vi "Copy exp data.vi"(8 "error in (no error)":errorcluster, 9 "selected wavelengths":dbl[](array[numeric])=[550.0, 640.0, 680.0, 720.0, 780.0, 800.0], 10 "ItemTag":string, 11 "Control-Client in":refnum<class "Control-Client.lvclass">) -> (0 "error out":errorcluster, 3 "Control-Client out":refnum<class "Control-Client.lvclass">)   [LabVIEW 2018, in "Control-Client.lvclass"]
uses:
  Control-Client.lvclass
  C:/Users/Sergey Denisov/Documents/REPS/TRANCON/Classes/GeneralFunctionality/GeneralFunctionality.lvclass
  GeneralFunctionality/GeneralFunctionality.lvclass/GeneralFunctionality.ctl
  Config/Config.lvclass
  Experiments/Experiment.lvclass
  GeneralFunctionality/GeneralFunctionality.lvclass
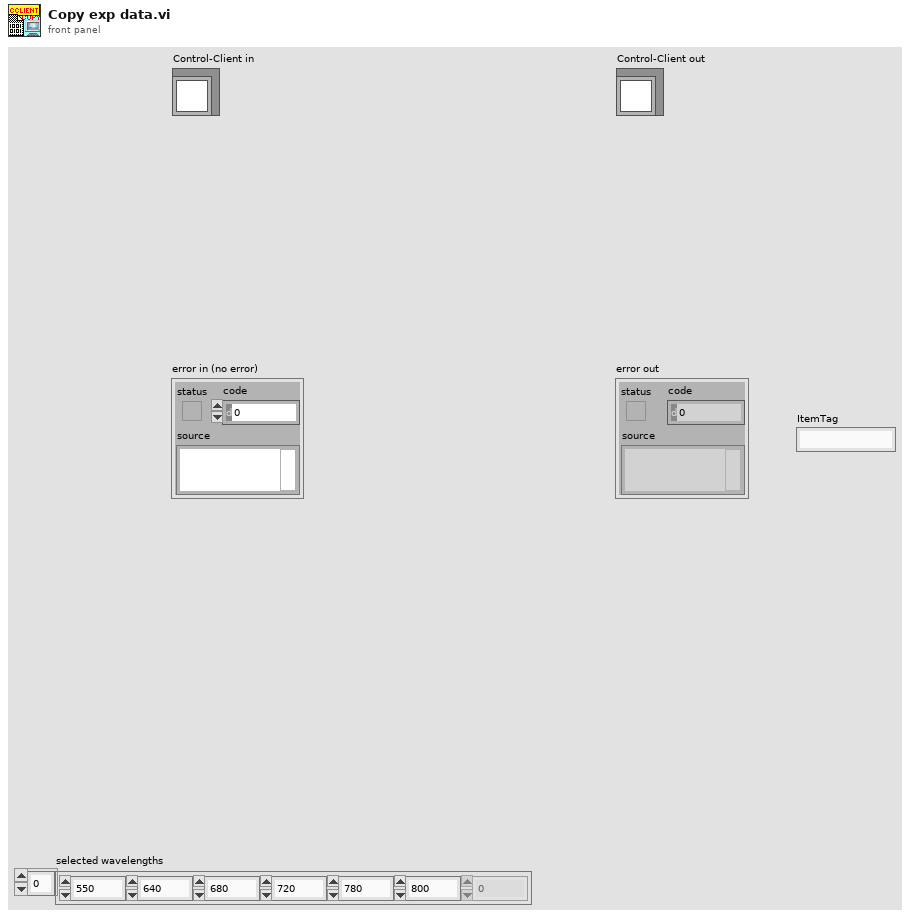
[diagram p1: front panel]
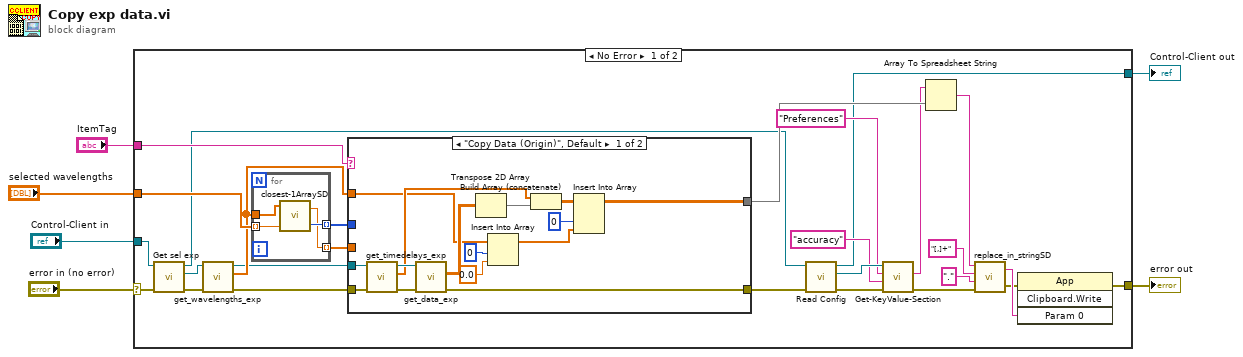
[diagram p0: block diagram]
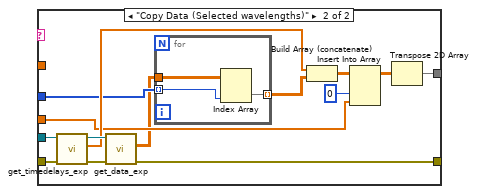
[diagram p2: hidden frame]
diagram:
  n1 = case shown="No Error" "error in (no error)" {
    selector: "error in (no error)" -> [w26 w71]
    tunnel: [w8 w71] -> w5
    tunnel: [w7 w70] -> w3
    tunnel: "Control-Client in" -> [w18 w70]
    tunnel: "selected wavelengths" -> [w27 _]
    tunnel: "ItemTag" -> [w19 _]
    frame No Error {
      n2 = call "Get sel exp.vi"("error in (no error)"=w26, "Control-Client in"=w18) -> ("error out"=w22:errorcluster, "Sel experiment"=w24:refnum<class "Experiment.lvclass">, "Control-Client out"=w10:refnum<class "Control-Client.lvclass">)  [unwired: 7 in]
      n3 = call "get_wavelengths_exp.vi"("error in (no error)"=w22, "Experiment.lvclass in"=w24) -> ("error out"=w21:errorcluster, "wavelengths"=w23:dbl[], "Experiment.lvclass out"=w20:refnum<class "Experiment.lvclass">)  [unwired: 7 in]
      n4 = for {
        tunnel: w27 -> [w36] mode=indexing
        tunnel: w23 -> [w37]
        tunnel: [w35] -> w32 mode=indexing
        tunnel: [w34] -> w25 mode=indexing
        n5 = call "closest-1ArraySD.vi"("desired element"=w36, "1D Array"=w37) -> ("closest index"=w35:i32, "closest element"=w34:dbl)  [unwired: 1 in]
      }
      n6 = case shown="\"Copy Data (Origin)\", Default" w19 {
        tunnel: [w43 w55] -> w28
        tunnel: [w38 w60] -> w17
        tunnel: w25 -> [_ w61]
        tunnel: w32 -> [_ w59]
        tunnel: w20 -> [w41 w54]
        tunnel: w21 -> [w40 w53]
        tunnel: w23 -> [w39 _]
        frame "Copy Data (Origin)", Default {
          n7 = call "get_timedelays_exp.vi"("error in (no error)"=w40, "Experiment.lvclass in"=w41) -> ("error out"=w42:errorcluster, "timedelays"=w51:dbl[], "Experiment.lvclass out"=w52:refnum<class "Experiment.lvclass">)  [unwired: 7 in]
          n8 = call "get_data_exp.vi"("error in (no error)"=w42, "Experiment.lvclass in"=w52) -> ("error out"=w38:errorcluster, "Data"=w50:sgl[][])  [unwired: 7 in, 1 out]
          n9 = Transpose 2D Array(2D array=w50) -> (transposed array=w49:sgl[][])
          n10 = Insert Into Array(array=w39, index=0, new element=0.0 ("new element/subarray")) -> (w44:dbl[])
          n11 = Build Array (concatenate)(w51, w49) -> (w46:dbl[][])
          n12 = Insert Into Array(array=w46, index (col)=0 ("disabled index (col)"), new element=w44) -> (w43:dbl[][])  [unwired: 1 in]
        }
        frame "Copy Data (Selected wavelengths)" {
          n13 = call "get_timedelays_exp.vi"("error in (no error)"=w53, "Experiment.lvclass in"=w54) -> ("error out"=w62:errorcluster, "timedelays"=w65:dbl[], "Experiment.lvclass out"=w66:refnum<class "Experiment.lvclass">)  [unwired: 7 in]
          n14 = call "get_data_exp.vi"("error in (no error)"=w62, "Experiment.lvclass in"=w66) -> ("error out"=w60:errorcluster, "Data"=w58:sgl[][])  [unwired: 7 in, 1 out]
          n15 = for {
            tunnel: w58 -> [w69]
            tunnel: w59 -> [w67] mode=indexing
            tunnel: [w68] -> w57 mode=indexing
            n16 = Index Array(array=w69, index (col)=w67) -> (element=w68:sgl[])  [unwired: 1 in]
          }
          n17 = Build Array (concatenate)(w65, w57) -> (w64:dbl[][])
          n18 = Insert Into Array(array=w64, index (col)=0 ("disabled index (col)"), new element=w61) -> (w56:dbl[][])  [unwired: 1 in]
          n19 = Transpose 2D Array(2D array=w56) -> (transposed array=w55:dbl[][])
        }
      }
      n20 = call "Read Config.vi"("error in (no error)"=w17, "GeneralFunctionality en entrée"=w10) -> ("error out"=w15:errorcluster, "Config.lvclass"=w14:refnum<class "Config.lvclass">, "GeneralFunctionality en sortie"=w7:refnum<class "Control-Client.lvclass">)  [unwired: 7 in]
      n21 = call-dynamic "Get-KeyValue-Section.vi"("error in (no error)"=w15, "Key"="accuracy", "Section"="Preferences", "Config in"=w14) -> ("error out"=w9:errorcluster, "Value"=w11:string)  [unwired: 5 in, 1 out]
      n22 = Array To Spreadsheet String(array=w28, 3:w11) -> (spreadsheet string=w31:string)  [unwired: 1 in]
      n23 = call "replace_in_stringSD.vi"("error in (no error)"=w9, "replaced to.."=".", "characters to replace"="[,]+", "input string"=w31) -> ("error out"=w16:errorcluster, "output string"=w33:string)
      n24 = invoke class="App" method="Clipboard.Write"(error in=w16, "Param 0"=w33) -> (error out=w8:errorcluster)  [unwired: 2 in, 3 out]
    }
    frame Error {
    }
  }
  "error out" <- w5
  "Control-Client out" <- w3
